vi "ep_Get Spectra Points In Window.vi"(8 "error in (no error)":errorcluster, 9 "points of half window length":u8=1, 10 "sideband center frequency":dbl, 11 "all spectra points":cluster{"frequency":dbl[], "magnitude":dbl[]}) -> (0 "error out":errorcluster, 3 "spectra points in window":cluster{"frequency":dbl[], "magnitude":dbl[]})   [LabVIEW 2014, in "NI_EP_Motor Monitoring.lvlib"]
uses:
  <vilib>/addons/Electrical Power/Motor Monitoring/NI_EP_Motor Monitoring.lvlib
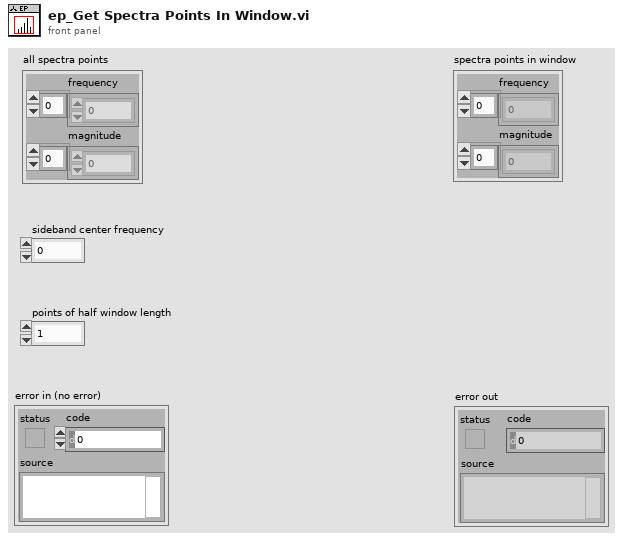
[diagram p1: front panel]
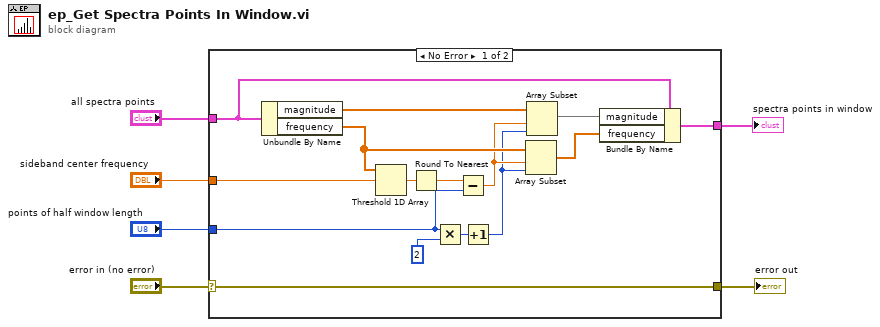
[diagram p0: block diagram]
diagram:
  n1 = case shown="No Error" "error in (no error)" {
    selector: "error in (no error)" -> [w8 w22]
    tunnel: [w8 w22] -> w5
    tunnel: "all spectra points" -> [w15 _]
    tunnel: "sideband center frequency" -> [w21 _]
    tunnel: "points of half window length" -> [w10 _]
    tunnel: [w12 _] -> w1
    frame No Error {
      n2 = Unbundle By Name(w15) -> ("magnitude"=w20:dbl[], "frequency"=w19:dbl[])
      n3 = Threshold 1D Array(2:w21, 3:w19) -> (0:w11:dbl)  [unwired: 1 in]
      n4 = Round To Nearest(number=w11) -> (nearest integer value=w7:dbl)
      n5 = Multiply(x=w10, y=2) -> (x*y=w16:i32)
      n6 = Subtract(x=w7, y=w10) -> (x-y=w17:dbl)
      n7 = Increment(x=w16) -> (x+1=w9:i32)
      n8 = Array Subset(array=w19, index=w17, length=w9) -> (w13:dbl[])
      n9 = Array Subset(array=w20, index=w17, length=w9) -> (w14:dbl[])
      n10 = Bundle By Name(cluster=w15, "magnitude"=w14, "frequency"=w13) -> (w12:cluster{"frequency":dbl[], "magnitude":dbl[]})
    }
    frame Error {
    }
  }
  "spectra points in window" <- w1
  "error out" <- w5
